vi "Cryostation.Get STR (All).vi"(8 "error in (no error)":errorcluster, 11 "instrument.Cryostation in":refnum<class "instrument.Cryostation.lvclass">) -> (0 "error out":errorcluster, 3 "instrument.Cryostation out":refnum<class "instrument.Cryostation.lvclass">)   [LabVIEW 2019, in "instrument.Cryostation.lvclass"]
uses:
  instrument.Cryostation.lvclass
  Typedefs/Cryostation.COM-STR--combo.ctl
  instrument.Cryostation.lvclass/instrument.Cryostation.ctl
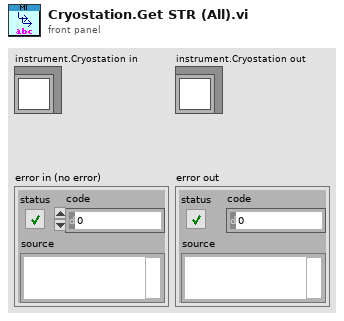
[diagram p1: front panel]
types:
  T1 = typedef "instrument.Cryostation.lvclass/Cryostation.COM-STR--combo.ctl" = string
  T2 = typedef "instrument.Cryostation.lvclass/Cryostation.getAll--cluster.ctl" = cluster{"Chamber Pressure (mTorr)":dbl, "Compressor Return Pressure (MPa)":dbl, "Compressor Supply Pressure (MPa)":dbl, "Compressor Speed (Hz)":dbl, "Cold Head Speed (Hz)":dbl, "Platform Heater Power (W)":dbl, "Platform Stability (K)":dbl, "Platform Temperature (K)":dbl, "Stage 1 Heater Power (W)":dbl, "Stage 1 Temperature (K)":dbl, "Stage 2 Heater Power (W)":dbl, "Stage 2 Temperature (K)":dbl, "Sample Stability (K)":dbl, "Sample Temperature (K)":dbl, "Temperature Set Point (K)":dbl, "User Stability (K)":dbl, "User Temperature (K)":dbl, "User Temperature Set Point (K)":dbl, "Alarm State":string, "Compressor Run State":string, "Case Valve State":string, "Idle State":string, "Nitrogen State":string, "Vent Valve State":string}
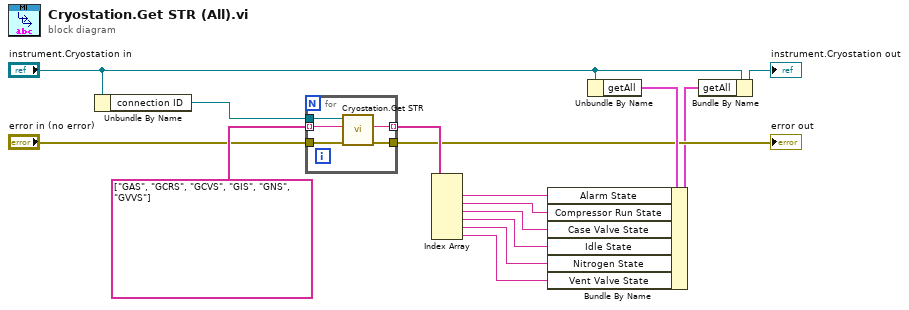
[diagram p0: block diagram]
diagram:
  n1 = Unbundle By Name("instrument.Cryostation in") -> ("connection ID"=w1:refnum<k5>)
  n2 = for {
    tunnel: w1 -> [w20]
    tunnel: T1[] ["GAS", "GCRS", "GCVS", "GIS", "GNS", "GVVS"] ("Array") -> [w19] mode=indexing
    tunnel: "error in (no error)" -> [w18]
    tunnel: [w17] -> w5
    tunnel: [w16] -> w6 mode=indexing
    n3 = call "Cryostation.Get STR.vi"("error in (no error)"=w18, "Command"=w19, "connection ID in"=w20) -> ("error out"=w17:errorcluster, "Response"=w16:string)  [unwired: 6 in, 1 out]
  }
  "error out" <- w5
  n4 = Index Array(array=w6) -> (element #1=w7:string, element #2=w8:string, element #3=w9:string, element #4=w10:string, element #5=w11:string, element #6=w12:string)  [unwired: 6 in]
  n5 = Unbundle By Name("instrument.Cryostation in") -> ("getAll"=w14:T2)
  n6 = Bundle By Name(cluster=w14, "Alarm State"=w7, "Compressor Run State"=w8, "Case Valve State"=w9, "Idle State"=w10, "Nitrogen State"=w11, "Vent Valve State"=w12) -> (w2:T2)
  n7 = Bundle By Name(cluster="instrument.Cryostation in", "getAll"=w2) -> (→"instrument.Cryostation out":refnum<class "instrument.Cryostation.lvclass">)
